vi "Fuld camera med gem og billede analyse.vi"() -> ()   [LabVIEW 2018]
uses:
  <vilib>/myRIO/Instrument Drivers/Onboard IO/PWM/typedefs/PWM Reference.ctl
  <vilib>/myRIO/Common/Instrument Driver Framework/Utilities/typedefs/myRIO Generic Hardware Reference.ctl
  <vilib>/myRIO/Common/Instrument Driver Framework/Utilities/typedefs/Hardware Version Enum.ctl
  <vilib>/myRIO/Common/Instrument Driver Framework/Utilities/typedefs/myRIO v1.0 Reference.ctl
  <vilib>/myRIO/Common/Instrument Driver Framework/Utilities/typedefs/Generic FPGA Reference.ctl
  <vilib>/myRIO/Common/Instrument Driver Framework/myRIO v1.0/PWM/typedefs/PWM Channels Enum.ctl
  <vilib>/myRIO/Instrument Drivers/Onboard IO/PWM/typedefs/PWM Configuration.ctl
  <vilib>/userdefined/High Color/nirio_resource_hc.ctl
  <vilib>/vision/Image Controls.llb/IMAQ Image.ctl
  <vilib>/myRIO/Common/Instrument Driver Framework/myRIO v1.0/PWM/vis/myRIO v1.1 Open PWM.vi
  <vilib>/myRIO/Common/Instrument Driver Framework/Utilities/vis/Validate Channels.vi
  <vilib>/myRIO/Common/Instrument Driver Framework/myRIO v1.0/PWM/vis/myRIO v1.0 Reserve PWM.vi
  <vilib>/myRIO/Common/Instrument Driver Framework/myRIO v1.0/UART/vis/myRIO v1.0 Close UART.vi
  <vilib>/myRIO/Common/Instrument Driver Framework/myRIO v1.0/PWM/vis/myRIO v1.0 Build MUX Configuration PWM.vi
  <vilib>/myRIO/Common/Instrument Driver Framework/myRIO v1.0/Resource Manager/vis/myRIO v1.0 Reserve Channel List.vi
  <vilib>/myRIO/Common/Instrument Driver Framework/myRIO v1.0/Resource Manager/vis/myRIO v1.0 Create Configuration List.vi
  <vilib>/myRIO/Common/Instrument Driver Framework/myRIO v1.0/Resource Manager/vis/myRIO v1.0 Reserve Channel.vi
  <vilib>/myRIO/Common/Instrument Driver Framework/myRIO v1.0/Resource Manager/vis/myRIO v1.0 Unreserve Channel.vi
  <vilib>/myRIO/Common/Instrument Driver Framework/myRIO v1.0/Resource Manager/vis/myRIO v1.0 Build Mutex Name.vi
  <vilib>/Utility/VariantDataType/GetNumericInfo.vi
  <vilib>/Utility/error.llb/Error Cluster From Error Code.vi
  <vilib>/myRIO/Common/Instrument Driver Framework/myRIO v1.0/myRIO v1.1 Open.vi
  <vilib>/myRIO/Common/Instrument Driver Framework/Utilities/vis/IO Manager.vi
  <vilib>/myRIO/Common/Instrument Driver Framework/Utilities/vis/Configuration Manager.vi
  <vilib>/myRIO/Common/Instrument Driver Framework/myRIO v1.0/Resource Manager/vis/myRIO v1.0 Configure IO.vi
  <vilib>/myRIO/Common/Instrument Driver Framework/myRIO v1.0/myRIO v1.0 Close.vi
  <vilib>/myRIO/Common/Instrument Driver Framework/myRIO v1.0/PWM/vis/myRIO v1.0 Write PWM.vi
  <vilib>/myRIO/Common/Instrument Driver Framework/Utilities/vis/FPGA Ref Manager.vi
  <vilib>/myRIO/Common/Instrument Driver Framework/myRIO v1.0/myRIO v1.0 Reset FPGA.vi
  <vilib>/myRIO/Common/Instrument Driver Framework/myRIO v1.0/IRQ/vis/myRIO v1.0 IRQ Info FGV.vi
  <vilib>/myRIO/Common/Instrument Driver Framework/myRIO v1.0/IRQ/vis/myRIO v1.0 Timer IRQ Info FGV.vi
  <vilib>/myRIO/Common/Instrument Driver Framework/myRIO v1.0/IRQ/vis/myRIO v1.0 ISR Agent.vi
  <vilib>/myRIO/Instrument Drivers/Onboard IO/PWM/vis/myRIO PWM Open.xnode
  <vilib>/myRIO/Instrument Drivers/Onboard IO/PWM/PWM.lvlib
  <vilib>/vision/driver/NI_Vision_Acquisition_Software.lvlib
  <vilib>/vision/NI_Vision_Development_Module.lvlib
  <vilib>/myRIO/Instrument Drivers/Utilities/Utilities.lvlib
panel:
  out "Image 6":T1(plugin-control)
  in  "Stop":bool
  out "Image 5":T1(plugin-control)
  out "Y 4":dbl[](array[numeric])
  out "X 4":dbl[](array[numeric])
  out "Antal isbjerg 4":i32
  out "logfile name":path
  in  "logfile base name":string="logfile"
  in  "Color Plane (Color Plane Extraction 1) 2":i32(ring)=1 items=["Red", "Green", "Blue", "Hue", "Saturation", "Luminance", "Value", "Intensity"]
  in  "Range (Threshold 1) 2":cluster{"Lower value":sgl, "Upper value":sgl}={"Lower value"=230.0, "Upper value"=255.0}
  in  "Structuring Element (Basic Morphology 1) 2":i32[][](array[numeric])=[[0, 1, 0], [1, 1, 1], [0, 1, 0]]
  in  "Number of Erosion (Advanced Morphology 1)":i32=12
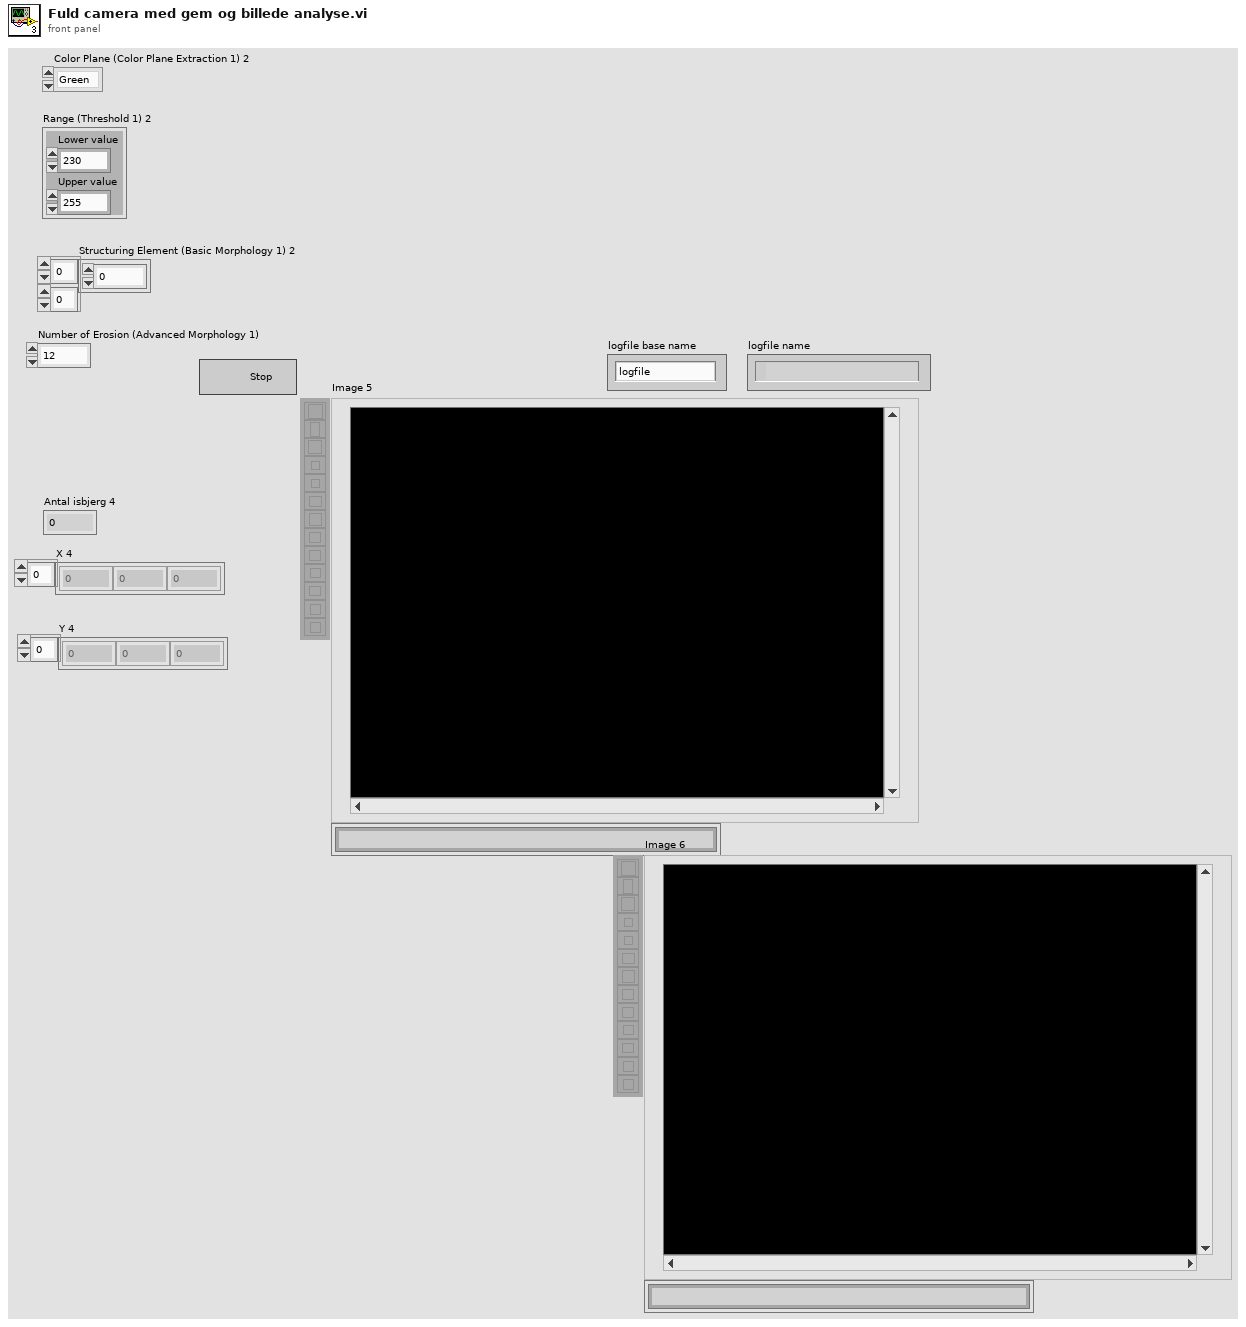
[diagram p1: front panel]
types:
  T1 = typedef "IMAQ Image.ctl" = refnum<image>
  T2 = typedef "nirio_resource_hc.ctl" = tag
  T3 = typedef "Hardware Version Enum.ctl" = enum16{"Unknown", "myRIO-1900", "myRIO-1950", "roboRIO", "NI ELVIS RIO CM", "ELVIS III"}
  T4 = enum32{"AutoM", "Close", "Dilate", "Erode", "Gradient", "Gradient out", "Gradient in", "Hit miss", "Open", "PClose", "POpen", "Thick", "Thin"}
  T5 = typedef "PWM.lvlib/PWM Reference.ctl" = cluster{"myRIO Reference":T6, "PWM Channels Enum":T9, "PWM Configuration":T10}
  T6 = typedef "myRIO Generic Hardware Reference.ctl" = cluster{"myRIO Model":T3, "myRIO Hardware Reference":T7}
  T7 = typedef "myRIO v1.0 Reference.ctl" = cluster{"Generic FPGA Reference":T8, "Allow multiple opens":bool}
  T8 = typedef "Generic FPGA Reference.ctl" = refnum<k20>
  T9 = typedef "PWM Channels Enum.ctl" = enum16{"Not Connected", "C/PWM0", "C/PWM1", "A/PWM0", "A/PWM1", "A/PWM2", "A/PWM3", "A/PWM4", "A/PWM5", "A/PWM6", "A/PWM7", "A/PWM8", "A/PWM9", "A/PWM10", "A/PWM11", "A/PWM12", "A/PWM13", "A/PWM14", "A/PWM15", "A/PWM16", "A/PWM17", "A/PWM18", "A/PWM19", "B/PWM0", "B/PWM1", "B/PWM2", "B/PWM3", "B/PWM4", "B/PWM5", "B/PWM6", "B/PWM7", "B/PWM8", "B/PWM9", "B/PWM10", "B/PWM11", "B/PWM12", "B/PWM13", "B/PWM14", "B/PWM15", "B/PWM16", "B/PWM17", "B/PWM18", "B/PWM19", "PWM/PWM0", "PWM/PWM1", "PWM/PWM2", "PWM/PWM3", "PWM/PWM4", "PWM/PWM5", "PWM/PWM6", "PWM/PWM7", "PWM/PWM8", "PWM/PWM9"}
  T10 = typedef "PWM.lvlib/PWM Configuration.ctl" = cluster{"Frequency":dbl, "Duty Cycle":dbl}
  T11 = typedef "Image Type" = u32
  T12 = typedef "IMAQdx.ctl" = refnum<k21>
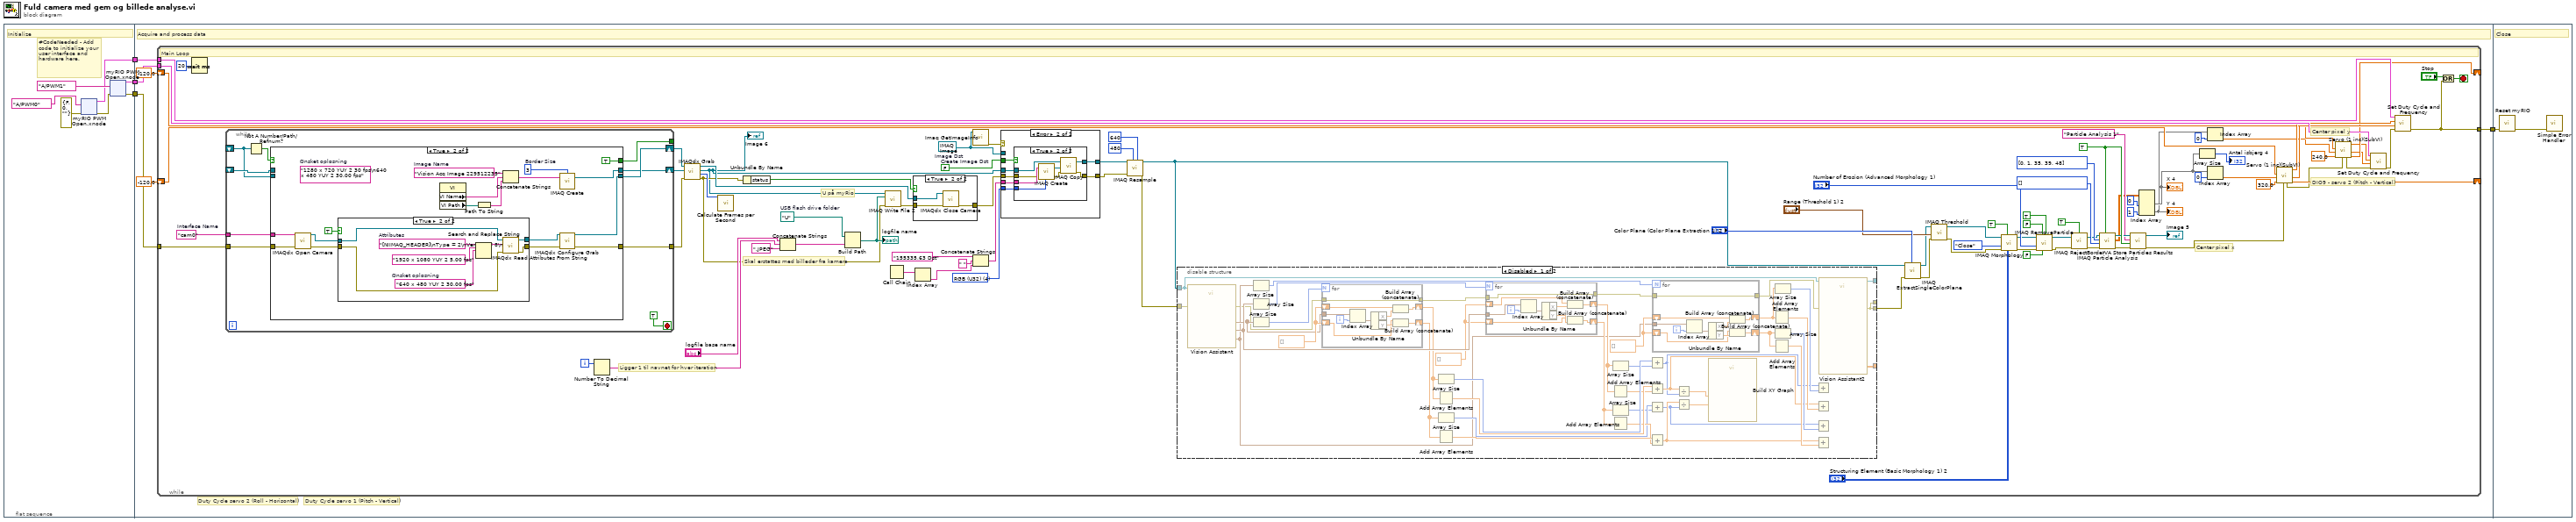
[diagram p0: block diagram]
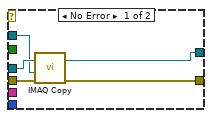
[diagram p6: hidden frame]
diagram:
  n1 = flat-sequence {
    tunnel: [w11] -> w4
    tunnel: [w10] -> w3
    tunnel: [w7] -> w2
    tunnel: w4 -> [w49]
    tunnel: w3 -> [w44]
    tunnel: w2 -> [w48]
    tunnel: [w47] -> w1
    tunnel: w1 -> [w284]
    frame #0 {
      # "#CodeNeeded - Add code to initialize your user interface and hardware here."
      # "Initialize"
      n2 = xnode "myRIO PWM Open.xnode"("error in (no error)"=errorcluster {"status"=FALSE, "code"=0, "source"=""} ("error in"), "Channel Name"=tag "A/PWM0") -> ("error out"=w5:errorcluster, "PWM Ref Out"=w7:T5)  [unwired: 1 in]
      n3 = xnode "myRIO PWM Open.xnode"("error in (no error)"=w5, "Channel Name"=tag "A/PWM1") -> ("error out"=w10:errorcluster, "PWM Ref Out"=w11:T5)  [unwired: 1 in]
    }
    frame #1 {
      # "Duty Cycle servo 2 (Roll - Horisontal)"
      # "Duty Cycle servo 1 (Pitch - Vertical)"
      # "Acquire and process data"
      n4 = while {
        tunnel: w49 -> [w141]
        tunnel: w48 -> [w140]
        tunnel: [w139] -> w47
        shift-right: [w99] -> _
        shift-left: -120.0 ("Duty Cycle servo 1 (Yaw - Horisontal)") -> [w103]
        shift-right: [w118] -> _
        shift-left: -120.0 ("Duty Cycle servo 1 (Yaw - Horisontal)") -> [w120]
        tunnel: w44 -> [w121]
        i -> [w88]
        stop <- w138 stop-if-true
        w66 = i32[] [] items=["Center of Mass X", "Center of Mass Y", "First Pixel X", "First Pixel Y", "Bounding Rect Left", "Bounding Rect Top", "Bounding Rect Right", "Bounding Rect Bottom", "Max Feret Diameter Start X", "Max Feret Diameter Start Y", "Max Feret Diameter End X", "Max Feret Diameter End Y", "Max Horiz. Segment Length Left", "Max Horiz. Segment Length Right", "Max Horiz. Segment Length Row", "-", "Bounding Rect Width", "Bounding Rect Height", "Bounding Rect Diagonal", "Perimeter", "Convex Hull Perimeter", "Holes' Perimeter", "Max Feret Diameter", "Equivalent Ellipse Major Axis", "Equivalent Ellipse Minor Axis", "Equivalent Ellipse Minor Axis (Feret)", "Equivalent Rect Long Side", "Equivalent Rect Short Side", "Equivalent Rect Diagonal", "Equivalent Rect Short Side (Feret)", "Average Horiz. Segment Length", "Average Vert. Segment Length", "Hydraulic Radius", "Waddel Disk Diameter", "-", "Area", "Holes' Area", "Particle & Holes' Area", "Convex Hull Area", "Image Area", "-", "Number of Holes", "Number of Horiz. Segments", "Number of Vert. Segments", "-", "Orientation", "Max Feret Diameter Orientation", "-", "% Area/Image Area", "% Area/(Particle & Holes' Area)", "Ratio of Equivalent Ellipse Axes", "Ratio of Equivalent Rect Sides", "-", "Elongation Factor", "Compactness Factor", "Heywood Circularity Factor", "Type Factor", "-", "Sum X", "Sum Y", "Sum XX", "Sum XY", "Sum YY", "Sum XXX", "Sum XXY", "Sum XYY", "Sum YYY", "-", "Moment of Inertia XX", "Moment of Inertia XY", "Moment of Inertia YY", "Moment of Inertia XXX", "Moment of Inertia XXY", "Moment of Inertia XYY", "Moment of Inertia YYY", "Norm. Moment of Inertia XX", "Norm. Moment of Inertia XY", "Norm. Moment of Inertia YY", "Norm. Moment of Inertia XXX", "Norm. Moment of Inertia XXY", "Norm. Moment of Inertia XYY", "Norm. Moment of Inertia YYY", "Hu Moment 1", "Hu Moment 2", "Hu Moment 3", "Hu Moment 4", "Hu Moment 5", "Hu Moment 6", "Hu Moment 7"] ("Real-World Measurements")
        w67 = i32[] [0, 1, 35, 39, 48] items=["Center of Mass X", "Center of Mass Y", "First Pixel X", "First Pixel Y", "Bounding Rect Left", "Bounding Rect Top", "Bounding Rect Right", "Bounding Rect Bottom", "Max Feret Diameter Start X", "Max Feret Diameter Start Y", "Max Feret Diameter End X", "Max Feret Diameter End Y", "Max Horiz. Segment Length Left", "Max Horiz. Segment Length Right", "Max Horiz. Segment Length Row", "-", "Bounding Rect Width", "Bounding Rect Height", "Bounding Rect Diagonal", "Perimeter", "Convex Hull Perimeter", "Holes' Perimeter", "Max Feret Diameter", "Equivalent Ellipse Major Axis", "Equivalent Ellipse Minor Axis", "Equivalent Ellipse Minor Axis (Feret)", "Equivalent Rect Long Side", "Equivalent Rect Short Side", "Equivalent Rect Diagonal", "Equivalent Rect Short Side (Feret)", "Average Horiz. Segment Length", "Average Vert. Segment Length", "Hydraulic Radius", "Waddel Disk Diameter", "-", "Area", "Holes' Area", "Particle & Holes' Area", "Convex Hull Area", "Image Area", "-", "Number of Holes", "Number of Horiz. Segments", "Number of Vert. Segments", "-", "Orientation", "Max Feret Diameter Orientation", "-", "% Area/Image Area", "% Area/(Particle & Holes' Area)", "Ratio of Equivalent Ellipse Axes", "Ratio of Equivalent Rect Sides", "-", "Elongation Factor", "Compactness Factor", "Heywood Circularity Factor", "Type Factor", "-", "Sum X", "Sum Y", "Sum XX", "Sum XY", "Sum YY", "Sum XXX", "Sum XXY", "Sum XYY", "Sum YYY", "-", "Moment of Inertia XX", "Moment of Inertia XY", "Moment of Inertia YY", "Moment of Inertia XXX", "Moment of Inertia XXY", "Moment of Inertia XYY", "Moment of Inertia YYY", "Norm. Moment of Inertia XX", "Norm. Moment of Inertia XY", "Norm. Moment of Inertia YY", "Norm. Moment of Inertia XXX", "Norm. Moment of Inertia XXY", "Norm. Moment of Inertia XYY", "Norm. Moment of Inertia YYY", "Hu Moment 1", "Hu Moment 2", "Hu Moment 3", "Hu Moment 4", "Hu Moment 5", "Hu Moment 6", "Hu Moment 7"] ("Pixel Measurements")
        w64 = TRUE ("Connectivity 4/8 (8)")
        w87 = path "U:/"  # USB flash drive folder
        w127 = "cam0"  # Interface Name
        w137 = T1 refnum  # Image Dst
        w129 = T11 4 items=["Grayscale (U8)", "Grayscale (I16)", "Grayscale (SGL)", "Complex (CSG)", "RGB (U32)", "HSL (U32)", "RGB (U64)", "Grayscale (U16)"] ("Image Dst Type")
        w135 = FALSE  # Create Image Dst
        # "U på myRio"
        # "Ligger 1 til navnet for hver iteration"
        # "Skal erstattes med billeder fra kamera"
        # "Center pixel y"
        # "Center pixel x"
        # "DIO9 - servo 2 (Pitch - Vertical)"
        # "Main Loop"
        n5 = Wait (ms)(milliseconds to wait=u32 20) -> ()  [unwired: 1 out]
        n6 = while "While Loop_template0" {
          shift-right: [w231] -> w122
          shift-left: _ -> [w224]
          tunnel: [w230] -> w128
          tunnel: w121 -> [w229]
          shift-right: [w227] -> w123
          shift-left: _ -> [w226]
          tunnel: w127 -> [w225]
          tunnel: [w222] -> _
          stop <- TRUE ("_template0") stop-if-true
          n7 = Not A Number/Path/Refnum?(number/path/refnum=w224) -> (NaN/Path/Refnum?=w223:bool)
          n8 = case "Case Structure_template0" shown="True" w223 {
            tunnel: [w234 w250] -> w231
            tunnel: w224 -> [w234 _]
            tunnel: [w233 w249] -> w230
            tunnel: w229 -> [w233 w251]
            tunnel: [w232 w248] -> w227
            tunnel: w226 -> [w232 _]
            tunnel: w225 -> [_ w239]
            tunnel: [_ TRUE] -> w222
            frame False {
            }
            frame True {
              (unwired) "1280 x 720 YUY 2 30 fps\n640 x 480 YUY 2 30.00 fps"  # Ønsket opløsning
              w236 = 3  # Border Size
              w243 = "Vision Acq Image 229512235"  # Image Name
              n9 = call <vilib>:"IMAQdx Open Camera.vi"("error in"=w251, "Session In"=w239) -> ("error out"=w241:errorcluster, "Session Out"=w242:T12)  [unwired: 1 in, 7 out]
              n10 = case shown="True" TRUE ("Init Attributes") {
                tunnel: w242 -> [w253 w261]
                tunnel: w241 -> [w252 w260]
                tunnel: [w253 w259] -> w235
                tunnel: [w252 w258] -> w240
                frame False {
                }
                frame True {
                  w254 = "640 x 480 YUY 2 30.00 fps"  # Ønsket opløsning
                  w257 = "[NIIMAQ_HEADER]\nType = 2\nVersion = 8\n\n[CAMERA_DATA]\nAcquisitionAttributes::Bayer::Algorithm = \"Bilinear\"\nAcquisitionAttributes::Bayer::GainB = \"1\"\nAcquisitionAttributes::Bayer::GainG = \"1\"\nAcquisitionAttributes::Bayer::GainR = \"1\"\nAcquisitionAttributes::Bayer::Pattern = \"Use hardware value\"\nAcquisitionAttributes::BitsPerPixel = \"Use hardware value\"\nAcquisitionAttributes::HardwareMaximumQueuedBufferCount = \"1000\"\nAcquisitionAttributes::HardwareRequeueBufferListThreshold = \"50\"\nAcquisitionAttributes::IgnoreFirstFrame = \"false\"\nAcquisitionAttributes::ImageDecoderCopyMode = \"Auto\"\nAcquisitionAttributes::OutputImageType = \"Auto\"\nAcquisitionAttributes::OverwriteMode = \"Get Newest\"\nAcquisitionAttributes::PixelSignedness = \"Use hardware value\"\nAcquisitionAttributes::ReceiveTimestampMode = \"None\"\nAcquisitionAttributes::ShiftPixelBits = \"false\"\nAcquisitionAttributes::SwapPixelBytes = \"false\"\nAcquisitionAttributes::Timeout = \"5000\"\nAcquisitionAttributes::VideoMode = \"1920 x 1080 YUY 2 5.00 fps\"\nCameraAttributes::BacklightCompensation::Mode = \"Manual\"\nCameraAttributes::BacklightCompensation::Value = \"0\"\nCameraAttributes::Brightness::Mode = \"Manual\"\nCameraAttributes::Brightness::Value = \"168\"\nCameraAttributes::Contrast::Mode = \"Manual\"\nCameraAttributes::Contrast::Value = \"5\"\nCameraAttributes::Exposure::Mode = \"AutoAperaturePriority\"\nCameraAttributes::Focus::Mode = \"Auto\"\nCameraAttributes::Pan::Mode = \"Manual\"\nCameraAttributes::Pan::Value = \"0\"\nCameraAttributes::PowerLineFrequency::Mode = \"60Hz\"\nCameraAttributes::Saturation::Mode = \"Manual\"\nCameraAttributes::Saturation::Value = \"103\"\nCameraAttributes::Sharpness::Mode = \"Manual\"\nCameraAttributes::Sharpness::Value = \"25\"\nCameraAttributes::Tilt::Mode = \"Manual\"\nCameraAttributes::Tilt::Value = \"0\"\nCameraAttributes::WhiteBalance::Mode = \"Auto\"\nCameraAttributes::Zoom::Mode = \"Manual\"\nCameraAttributes::Zoom::Value = \"0\"\n"  # Attributes
                  n11 = Search and Replace String(input string=w257, search string="1920 x 1080 YUY 2 5.00 fps", replace string=w254) -> (result string=w255:string)  [unwired: 5 in, 3 out]
                  n12 = call <vilib>:"IMAQdx Read Attributes From String.vi"("error in"=w260, "Attributes String In"=w255, "Session In"=w261) -> ("error out"=w258:errorcluster, "Session Out"=w259:T12)  [unwired: 7 out]
                }
              }
              n13 = property class="VI"() -> ("VI Name"=w246:string, "VI Path"=w247:path)  [unwired: 2 in, 2 out]
              n14 = Path To String(path=w247) -> (string=w245:string)
              n15 = Concatenate Strings(w243, w246, w245) -> (w244:string)
              n16 = call "IMAQ Create"("Border Size"=w236, "Image Name"=w244) -> ("New Image"=w248:T1)  [unwired: 2 in, 2 out]
              n17 = call <vilib>:"IMAQdx Configure Grab.vi"("error in"=w240, "Session In"=w235) -> ("error out"=w249:errorcluster, "Session Out"=w250:T12)  [unwired: 8 out]
            }
          }
        }
        n18 = Number To Decimal String(number=w88) -> (decimal integer string=w92:string)  [unwired: 1 in]
        n19 = call <vilib>:"IMAQdx Grab.vi"("error in"=w128, "Image In"=w123, "Session In"=w122) -> ("error out"=w90:errorcluster, "Buffer Number Out"=w126:u32, "Image Out"=w50:T1, "Session Out"=w125:T12)  [unwired: 1 in, 4 out]
        "Image 6" <- w50
        n20 = call <vilib>:"Calculate Frames per Second.vi"("Buffer Number"=w126) -> ()  [unwired: 2 in, 9 out]
        n21 = Unbundle By Name(w90) -> ("status"=w112:bool)
        n22 = Concatenate Strings "Concatenate Strings"("logfile base name", w92, ".JPEG" ("string")) -> (w94:string)
        n23 = Build Path(base path=w87, name or relative path=w94) -> (appended path=w95:path)
        "logfile name" <- w95
        n24 = call-poly "IMAQ Write File 2"("error in (no error)"=w90, "File Path"=w95, "Image"=w50) -> ("error out"=w89:errorcluster)  [unwired: 7 in, 1 out]
        n25 = Call Chain() -> (call chain=w134:string[])
        n26 = case "Case Structure_template1" shown="True" w112 {
          tunnel: [w218 w220] -> w124
          tunnel: w89 -> [w218 w221]
          tunnel: w125 -> [_ w219]
          frame False {
          }
          frame True {
            n27 = call <vilib>:"IMAQdx Close Camera.vi"("error in"=w221, "Session In"=w219) -> ("error out"=w220:errorcluster)  [unwired: 9 out]
          }
        }
        n28 = Index Array(array=w134) -> (element=w132:string)  [unwired: 1 in]
        n29 = call "Imaq GetImageInfo"("Image"=w137) -> ("error out"=w136:errorcluster)  [unwired: 1 in, 9 out]
        n30 = Concatenate Strings("155335,63 Dst" ("Image Dst Name"), " ", w132) -> (w130:string)
        n31 = case shown="Error" w136 {
          tunnel: [w266 w270] -> w53
          tunnel: [w265 w269] -> w52
          tunnel: w50 -> [w264 w271]
          tunnel: w124 -> [w263 w267]
          tunnel: w137 -> [w262 _]
          tunnel: w130 -> [_ w273]
          tunnel: w129 -> [_ w272]
          tunnel: w135 -> [_ w268]
          frame No Error {
            n32 = call "IMAQ Copy"("error in (no error)"=w263, "Image Dst"=w262, "Image Src"=w264) -> ("error out"=w265:errorcluster, "Image Dst Out"=w266:T1)  [unwired: 3 out]
          }
          frame Error {
            n33 = case shown="True" w268 {
              tunnel: w273 -> [_ w283]
              tunnel: w272 -> [_ w282]
              tunnel: w271 -> [w275 w280]
              tunnel: [w275 w279] -> w270
              tunnel: [w274 w278] -> w269
              tunnel: w267 -> [w274 w276]
              frame False {
              }
              frame True {
                n34 = call "IMAQ Create"("Image Name"=w283, "Image Type"=w282, "error in (no error)"=w276) -> ("New Image"=w281:T1, "error out"=w277:errorcluster)  [unwired: 1 in, 1 out]
                n35 = call "IMAQ Copy"("error in (no error)"=w277, "Image Dst"=w281, "Image Src"=w280) -> ("error out"=w278:errorcluster, "Image Dst Out"=w279:T1)  [unwired: 3 out]
              }
            }
          }
        }
        n36 = call "IMAQ Resample"("X Resolution"=u32 640 ("Width"), "Y Resolution"=u32 480 ("Height"), "error in (no error)"=w52, "Image Src"=w53) -> ("error out"=w51:errorcluster, "Image Dst Out"=w56:T1)  [unwired: 6 in]
        n37 = disable-structure shown="Disabled" {
          disable-tunnel: w51 -> [w187 _]
          disable-tunnel: w56 -> [w145 _]
          disable-tunnel: [w144 _] -> _
          disable-tunnel: [w143 _] -> _
          disable-tunnel: [w142 _] -> _
          disable-tunnel: [w142 _] -> w59
          frame Disabled {
            w167 = dbl[] []
            w180 = dbl[] []
            w184 = dbl[] []
            n38 = call "Vision Assistant"("Image In"=w145, "error in"=w187) -> ("Feature Points Coordinates (Feature Detection 3)"=w165:cluster{"X":dbl, "Y":dbl}[], "Feature Points Coordinates (Feature Detection 1)"=w169:cluster{"X":dbl, "Y":dbl}[], "Feature Points Coordinates (Feature Detection 2)"=w185:cluster{"X":dbl, "Y":dbl}[], "error out"=w159:errorcluster)  [unwired: 21 in, 1 out]
            n39 = Array Size(array=w165) -> (size(s)=w166:i32)
            n40 = Array Size(array=w185) -> (size(s)=w186:i32)
            n41 = Array Size(array=w169) -> (size(s)=w181:i32)
            n42 = for {
              N: w181 -> [_]
              shift-right: [w205] -> w179
              shift-left: w180 -> [w200]
              shift-right: [w204] -> w178
              shift-left: w180 -> [w201]
              tunnel: w169 -> [w199]
              tunnel: w159 -> [w198]
              tunnel: [w198] -> w158
              i -> [w207]
              n43 = Index Array(array=w199, index=w207) -> (element=w206:cluster{"X":dbl, "Y":dbl})
              n44 = Unbundle By Name(w206) -> ("X"=w203:dbl, "Y"=w202:dbl)
              n45 = Build Array (concatenate)(w200, w203) -> (w205:dbl[])
              n46 = Build Array (concatenate)(w201, w202) -> (w204:dbl[])
            }
            n47 = Add Array Elements(numeric array=w179) -> (sum=w175:dbl)
            n48 = Add Array Elements(numeric array=w178) -> (sum=w173:dbl)
            n49 = Array Size(array=w179) -> (size(s)=w177:i32)
            n50 = Array Size(array=w178) -> (size(s)=w171:i32)
            n51 = for {
              N: w186 -> [_]
              shift-right: [w215] -> w183
              shift-left: w184 -> [w210]
              shift-right: [w214] -> w182
              shift-left: w184 -> [w211]
              tunnel: w185 -> [w209]
              tunnel: w158 -> [w208]
              tunnel: [w208] -> w157
              i -> [w217]
              n52 = Index Array(array=w209, index=w217) -> (element=w216:cluster{"X":dbl, "Y":dbl})
              n53 = Unbundle By Name(w216) -> ("X"=w213:dbl, "Y"=w212:dbl)
              n54 = Build Array (concatenate)(w210, w213) -> (w215:dbl[])
              n55 = Build Array (concatenate)(w211, w212) -> (w214:dbl[])
            }
            n56 = Add Array Elements(numeric array=w183) -> (sum=w174:dbl)
            n57 = Add Array Elements(numeric array=w182) -> (sum=w172:dbl)
            n58 = Array Size(array=w183) -> (size(s)=w176:i32)
            n59 = Array Size(array=w182) -> (size(s)=w170:i32)
            n60 = Add(x=w177, y=w176) -> (x+y=w151:i32)
            n61 = Add(x=w175, y=w174) -> (x+y=w152:dbl)
            n62 = Add(x=w171, y=w170) -> (x+y=w149:i32)
            n63 = Add(x=w173, y=w172) -> (x+y=w150:dbl)
            n64 = for {
              N: w166 -> [_]
              shift-right: [w195] -> w168
              shift-left: w167 -> [w190]
              shift-right: [w194] -> w161
              shift-left: w167 -> [w191]
              tunnel: w165 -> [w189]
              tunnel: w157 -> [w188]
              tunnel: [w188] -> w156
              i -> [w197]
              n65 = Index Array(array=w189, index=w197) -> (element=w196:cluster{"X":dbl, "Y":dbl})
              n66 = Unbundle By Name(w196) -> ("X"=w193:dbl, "Y"=w192:dbl)
              n67 = Build Array (concatenate)(w190, w193) -> (w195:dbl[])
              n68 = Build Array (concatenate)(w191, w192) -> (w194:dbl[])
            }
            n69 = Divide(x=w152, y=w151) -> (x/y=w154:dbl)
            n70 = Divide(x=w150, y=w149) -> (x/y=w153:dbl)
            n71 = call "Build XY Graph"("Y Input"=w153, "X Input"=w154) -> ("XY Graph"=w155:cluster{"X":dbl[], "Y":dbl[]}[])  [unwired: 8 in, 1 out]
            n72 = Add Array Elements(numeric array=w168) -> (sum=w163:dbl)
            n73 = Add Array Elements(numeric array=w161) -> (sum=w162:dbl)
            n74 = Array Size(array=w168) -> (size(s)=w164:i32)
            n75 = Array Size(array=w161) -> (size(s)=w160:i32)
            n76 = Add(x=w151, y=w164) -> ()  [unwired: 1 out]
            n77 = Add(x=w152, y=w163) -> ()  [unwired: 1 out]
            n78 = Add(x=w149, y=w160) -> ()  [unwired: 1 out]
            n79 = Add(x=w150, y=w162) -> ()  [unwired: 1 out]
            n80 = call "Vision Assistant2"("Image In"=w145, "error in"=w156) -> ("Color Plane (Color Plane Extraction 1)"=w146:i32, "Range (Threshold 1)"=w147:cluster{"Lower value":sgl, "Upper value":sgl}, "Structuring Element (Basic Morphology 1)"=w148:i32[][], "Image Out"=w144:T1, "Particle Measurements (Pixels) (Particle Analysis 1)"=w143:dbl[][], "error out"=w142:errorcluster)  [unwired: 20 in]
          }
          frame Enabled {
          }
        }
        n81 = call "IMAQ ExtractSingleColorPlane"("Color Plane"="Color Plane (Color Plane Extraction 1) 2", "error in (no error)"=w59, "Image Src"=w56) -> ("error out"=w85:errorcluster, "Image Dst Out"=w83:T1)  [unwired: 1 in, 6 out]
        n82 = call "IMAQ Threshold"("error in (no error)"=w85, "Range"="Range (Threshold 1) 2", "Image Src"=w83) -> ("error out"=w82:errorcluster, "Image Dst Out"=w78:T1)  [unwired: 3 in, 4 out]
        n83 = call "IMAQ Morphology"("Structuring Element"="Structuring Element (Basic Morphology 1) 2", "Square/Hexa (Square)"=TRUE, "error in (no error)"=w82, "Operation"=T4."Close", "Image Src"=w78) -> ("error out"=w77:errorcluster, "Image Dst Out"=w72:T1)  [unwired: 2 in, 3 out]
        n84 = call "IMAQ RemoveParticle"("Connectivity 4/8 (8)"=TRUE, "Low Pass/High Pass (Low)"=FALSE, "Square/Hexa (Square)"=FALSE, "error in (no error)"=w77, "Number of Erosion"="Number of Erosion (Advanced Morphology 1)", "Image Src"=w72) -> ("error out"=w71:errorcluster, "Image Dst Out"=w69:T1)  [unwired: 1 in, 3 out]
        n85 = call "IMAQ RejectBorder"("error in (no error)"=w71, "Image Src"=w69, "Connectivity 4/8 (8)"=TRUE) -> ("error out"=w68:errorcluster, "Image Dst Out"=w65:T1)  [unwired: 1 in, 2 out]
        n86 = call "IMAQ Particle Analysis"("Connectivity 4/8 (8)"=w64, "error in (no error)"=w68, "Real-World Measurements"=w66, "Pixel Measurements"=w67, "Image"=w65) -> ("error out"=w61:errorcluster, "Particle Measurements (Pixels)"=w57:dbl[][], "Image Out (duplicate)"=w63:T1)  [unwired: 4 out]
        n87 = call <vilib>:"IVA Store Particles Results.vi"("error in (no error)"=w61, "Connectivity 4/8 (8)"=w64, "Step Name"="Particle Analysis 1", "Image in"=w63) -> ("error out"=w58:errorcluster, "Image dup"=→"Image 5":T1)  [unwired: 6 out]
        n88 = Index Array(array=w57, index (col) #1=0 ("index (col)"), index (col) #2=1 ("index (col)")) -> (element #1=w107:dbl[], element #2=w104:dbl[])  [unwired: 2 in]
        "Y 4" <- w104
        "X 4" <- w107
        n89 = Array Size(array=w107) -> (size(s)=→"Antal isbjerg 4":i32)
        n90 = Index Array(array=w104, index=0) -> (element=w96:dbl)
        n91 = Index Array(array=w107, index=0) -> (element=w106:dbl)
        n92 = call "Servo (1 inc)(SubVI).vi"("error constant 2"=w58, "Center pixel"=320.0 ("Center pixel 2"), "Pixel value"=w106, "Position."=w120) -> ("Position 2"=w118:dbl, "freq [Hz]"=w119:dbl, "Duty"=w117:dbl, "error constant"=w101:errorcluster)  [unwired: 3 in, 1 out]
        n93 = call "Servo (1 inc)(SubVI).vi"("error constant 2"=w101, "Center pixel"=240.0, "Pixel value"=w96, "Position."=w103) -> ("Position 2"=w99:dbl, "freq [Hz]"=w98:dbl, "Duty"=w97:dbl, "error constant"=w100:errorcluster)  [unwired: 3 in, 1 out]
        n94 = call <vilib>:"Set Duty Cycle and Frequency.vi"("error in (no error)"=w100, "Frequency [Hz]"=w98, "Duty Cycle"=w97, "PWM Ref In"=w141) -> ("error out"=w113:errorcluster)  [unwired: 5 in, 1 out]
        n95 = call <vilib>:"Set Duty Cycle and Frequency.vi"("error in (no error)"=w113, "Frequency [Hz]"=w119, "Duty Cycle"=w117, "PWM Ref In"=w140) -> ("error out"=w139:errorcluster)  [unwired: 5 in, 1 out]
        n96 = Or(x="Stop", y=w139) -> (x .or. y?=w138:bool)
      }
    }
    frame #2 {
      # "Close"
      n97 = call <vilib>:"Reset myRIO.vi"("error in (no error)"=w284) -> ("error out"=w285:errorcluster)  [unwired: 10 in]
      n98 = call <vilib>:"Simple Error Handler.vi"("error in (no error)"=w285) -> ()  [unwired: 4 in, 5 out]
    }
  }
